vi "Make Reset Laser Power Msg.vi"(9 "Shutter Enable":bool[](array[boolean]), 11 "Input Array":refnum<class "Message.lvclass">[](array[class])) -> (3 "Output Array":refnum<class "Message.lvclass">[](array[class]))   [LabVIEW 2023, in "Application.lvlib" / "Reset Laser Power Msg.lvclass"]
doc: "This VI sends the message to an actor."
uses:
  Reset Laser Power Msg.lvclass
  <vilib>/ActorFramework/Message/Message.lvclass
  Reset Laser Power Msg.lvclass/Reset Laser Power Msg.ctl
  C:/Program Files/National Instruments/LabVIEW 2023/vi.lib/ActorFramework/Message/Message.lvclass
  C:/FlashGordon/Development/Application Messages/Reset Laser Power Msg/Reset Laser Power Msg.lvclass
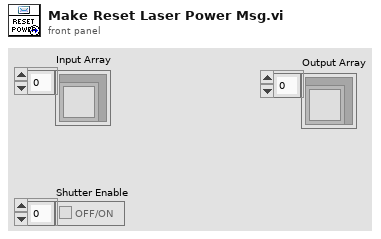
[diagram p1: front panel]
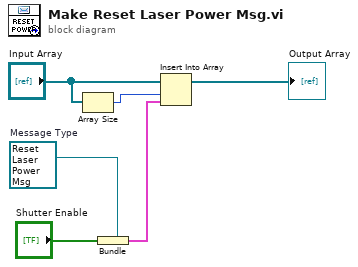
[diagram p0: block diagram]
diagram:
  w6 = refnum<class "Reset Laser Power Msg.lvclass"> refnum  # Message Type
  n1 = Array Size(array="Input Array") -> (size(s)=w1:i32)
  n2 = Bundle(cluster=w6, "Shutter Enable"="Shutter Enable") -> (w3:cluster{"Shutter Enable":bool[]})
  n3 = Insert Into Array(array="Input Array", index=w1, new element=w3) -> (→"Output Array":refnum<class "Message.lvclass">[])
